vi "Test_PackReturnMessageAdapter_ReturnToPacker_PackedMessageReceived.vi"(8 "error in (no error)":errorcluster, 11 "TestCase in":refnum<class "TestReturnMessageAdapter.lvclass">) -> (0 "error out":errorcluster, 3 "TestCase out":refnum<class "TestReturnMessageAdapter.lvclass">)   [LabVIEW 2017, in "TestReturnMessageAdapter.lvclass"]
uses:
  TestReturnMessageAdapter.lvclass
  <vilib>/ActorFramework/Batch Msg/Batch Msg.lvclass
  C:/Program Files (x86)/National Instruments/LabVIEW 2017/vi.lib/ActorFramework/Message/Message.lvclass
  <vilib>/ActorFramework/Message Queue/Message Queue.lvclass/Message Queue.ctl
  Source/ReturnMessageAdapter/ReturnMessageAdapter.lvclass/ReturnMessageAdapter.ctl
  <vilib>/ActorFramework/Message Enqueuer/Message Enqueuer.lvclass/Message Enqueuer.ctl
  <vilib>/ActorFramework/Message Dequeuer/Message Dequeuer.lvclass/Message Dequeuer.ctl
  <vilib>/ActorFramework/Message Enqueuer/Enqueue.vi
  <vilib>/ActorFramework/Message Priority Queue/Priority Enqueue.vi
  <vilib>/ActorFramework/Message Priority Queue/Priority Dequeue.vi
  Source/ReturnMessageAdapter/ReturnMessageAdapter.lvclass
  <vilib>/ActorFramework/Message Queue/Message Queue.lvclass
  <vilib>/ActorFramework/Message Dequeuer/Message Dequeuer.lvclass
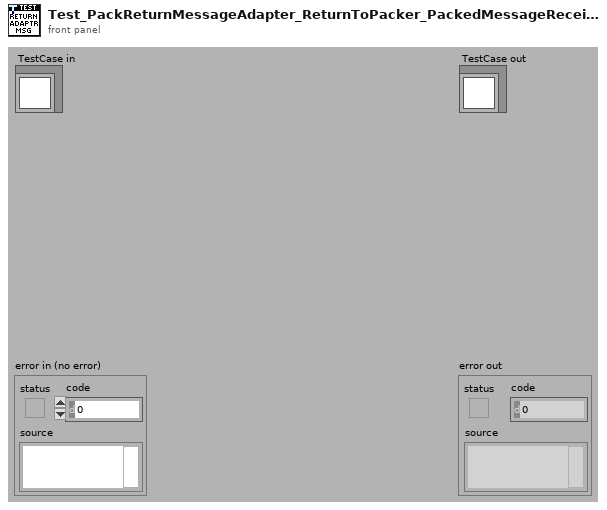
[diagram p1: front panel]
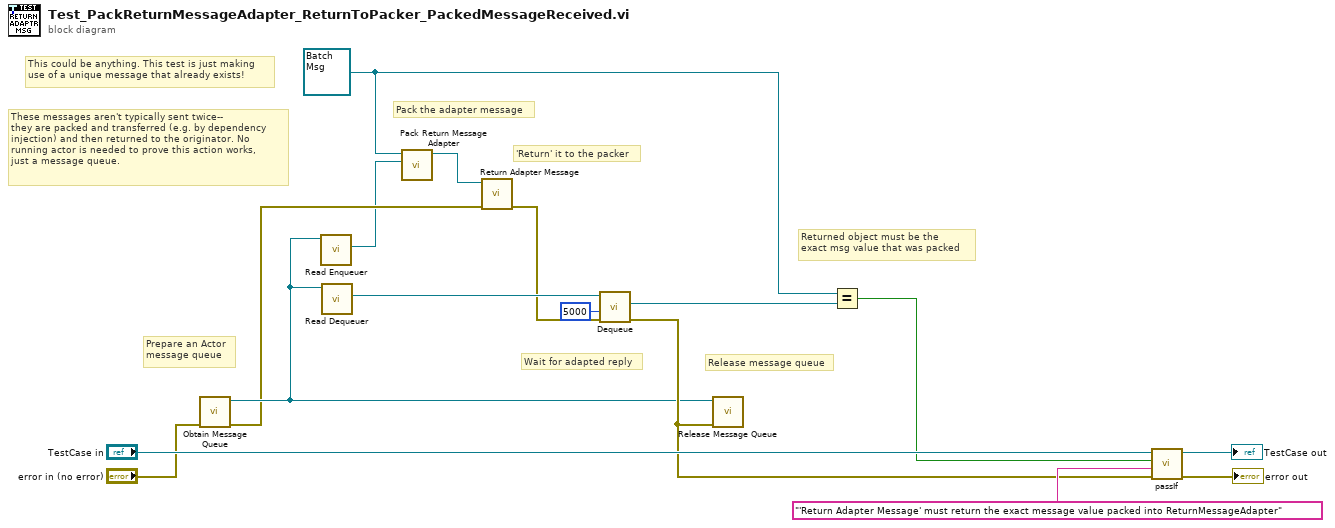
[diagram p0: block diagram]
diagram:
  w5 = refnum<class "Batch Msg.lvclass"> refnum ("Batch Msg")
  # "These messages aren't typically sent twice--\nthey are packed and transferred (e.g. by dependency\ninjection) and then returned to the originator. No\nrunning actor is needed to prove this action works,\njust a message queue."
  # "'Return' it to the packer"
  # "Pack the adapter message"
  # "This could be anything. This test is just making\nuse of a unique message that already exists!"
  # "Release message queue"
  # "Returned object must be the\nexact msg value that was packed"
  # "Prepare an Actor\nmessage queue"
  # "Wait for adapted reply"
  n1 = call <vilib>:"Obtain Message Queue.vi"("error in (no error)"="error in (no error)") -> ("error out"=w3:errorcluster, "Message Queue"=w6:refnum<class "Message Queue.lvclass">)  [unwired: 9 in]
  n2 = call <vilib>:"Read Enqueuer.vi"("Message Queue"=w6) -> ("Message Enqueuer"=w1:refnum<class "Message Enqueuer.lvclass">)  [unwired: 10 in]
  n3 = call <vilib>:"Read Dequeuer.vi"("Message Queue"=w6) -> ("Message Dequeuer"=w13:refnum<class "Message Dequeuer.lvclass">)  [unwired: 10 in]
  n4 = call "Pack Return Message Adapter.vi"("Return Enqueuer"=w1, "Return Message"=w5) -> ("ReturnMessageAdapter Out"=w4:refnum<class "ReturnMessageAdapter.lvclass">)  [unwired: 9 in]
  n5 = call "Return Adapter Message.vi"("error in (no error)"=w3, "ReturnMessageAdapter In"=w4) -> ("error out"=w2:errorcluster)  [unwired: 9 in]
  n6 = call <vilib>:"Dequeue.vi"("error in (no error)"=w2, "timeout in ms (-1)"=5000, "Message Dequeuer in"=w13) -> ("error out"=w7:errorcluster, "Message"=w10:refnum<class "Message.lvclass">)  [unwired: 4 in, 3 out]
  n7 = call <vilib>:"Release Message Queue.vi"("error in (no error)"=w7, "Message Queue"=w6) -> ()  [unwired: 8 in, 2 out]
  n8 = Equal?(x=w5, y=w10) -> (x = y?=w9:bool)
  n9 = call-dynamic "passIf.vi"("error in (no error)"=w7, "message (\"\")"="'Return Adapter Message' must return the exact message value packed into ReturnMessageAdapter" ("message (\"\")"), "pass"=w9, "TestCase in"="TestCase in") -> ("error out"=→"error out":errorcluster, "TestCase out"=→"TestCase out":refnum<class "TestReturnMessageAdapter.lvclass">)  [unwired: 6 in]
